vi "Frequency (1 Channel).vi"(8 "error in (no error)":errorcluster, 11 "waveform":waveform(dbl)) -> (0 "error out":errorcluster, 3 "frequency":dbl)   [LabVIEW 2013, in "NI_EP_Basic.lvlib"]
doc: "Calculates the fundamental frequency of a voltage or current signal. Wire data to the <B>waveform</B> input to determine the polymorphic instance to use or manually select the instance."
uses:
  <vilib>/addons/Electrical Power/Basic/NI_EP_Basic.lvlib
  <vilib>/measure/NI_MAPro.lvlib
  <vilib>/measure/NI_MABase.lvlib
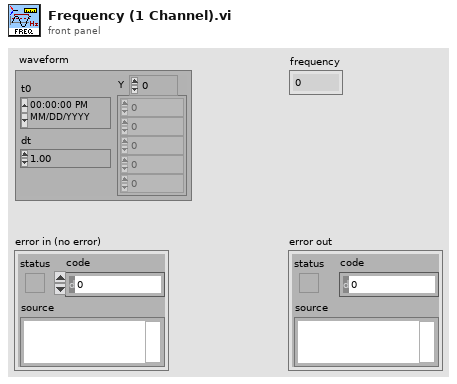
[diagram p1: front panel]
types:
  T1 = cluster{"approx freq. (optional)":dbl, "search (+/- % of Fsampl.)":dbl}
  T2 = enum32{"none", "input signal", "detected signal", "residual signal"}
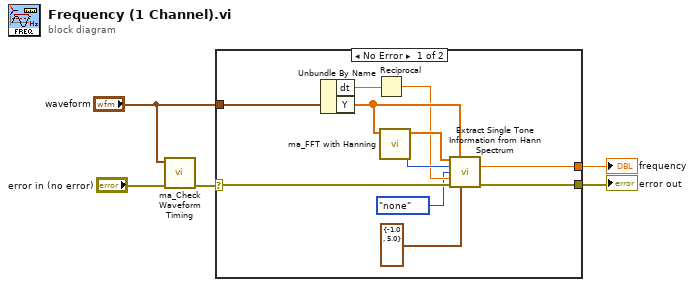
[diagram p0: block diagram]
diagram:
  n1 = call <vilib>:"ma_Check Waveform Timing.vi"("error in (no error)"="error in (no error)", "signal in"="waveform") -> ("error out"=w5:errorcluster)  [unwired: 1 in, 8 out]
  n2 = case shown="No Error" w5 {
    selector: w5 -> [w10 w17]
    tunnel: "waveform" -> [w16 _]
    tunnel: [w7 _] -> w4
    tunnel: [w6 w17] -> w1
    frame No Error {
      n3 = Unbundle By Name(w16) -> ("dt"=w12:dbl, "Y"=w15:dbl[])
      n4 = Reciprocal(x=w12) -> (1/x=w11:dbl)
      n5 = call <vilib>:"ma_FFT with Hanning.vi"("time signal data"=w15) -> ("FFT size"=w13:i32, "complex Hann spectrum"=w14:cdb[])  [unwired: 2 in, 7 out]
      n6 = call <vilib>:"Extract Single Tone Information from Hann Spectrum.vi"("complex spectrum in"=w14, "time signal in"=w15, "FFT size"=w13, "export mode"=T2."none", "sampling frequency"=w11, "error in"=w10, "advanced search"=T1 {"approx freq. (optional)"=-1.0, "search (+/- % of Fsampl.)"=5.0}) -> ("detected frequency"=w7:dbl, "error out"=w6:errorcluster)  [unwired: 7 out]
    }
    frame Error {
    }
  }
  "frequency" <- w4
  "error out" <- w1
